vi "_setEnvironmentId.vi"(4 "error in (no error)":errorcluster, 7 "EnvironmentID":i32=104) -> (0 "error out":errorcluster)   [LabVIEW 2017]
uses:
  lvStorage.dll
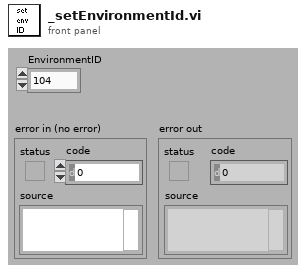
[diagram p1: front panel]
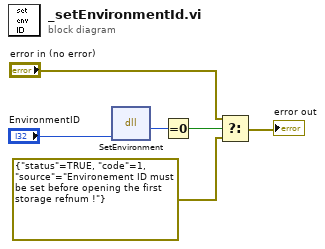
[diagram p0: block diagram]
diagram:
  n1 = dll-call lib="lvStorage.dll" fn="SetEnvironment"("EnvironmentID"="EnvironmentID") -> ("return type"=w5:i32)  [unwired: 4 in, 2 out]
  n2 = Equal To 0?(x=w5) -> (x = 0?=w3:bool)
  n3 = Select(t="error in (no error)", s=w3, f=errorcluster {"status"=TRUE, "code"=1, "source"="Environement ID must be set before opening the first storage refnum !"}) -> (s? t:f=→"error out":errorcluster)
